vi "reset arm.vi"   [LabVIEW 2018]
uses:
  ARM angles.vi
types:
  T1 = enum16{"shoulder", "elbow", "wrist", "base", "gripper"}
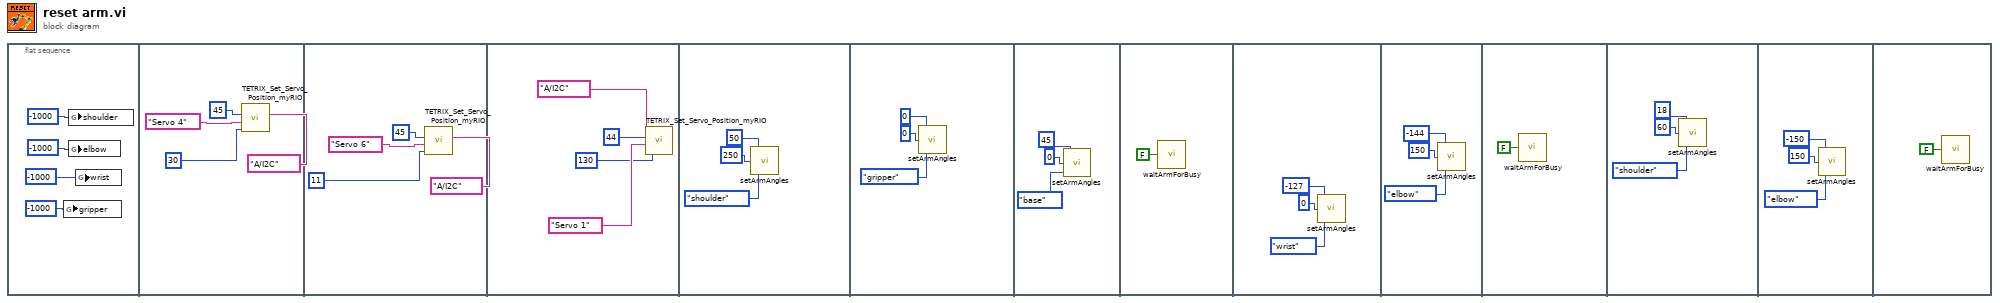
[diagram p0: block diagram]
diagram:
  n1 = flat-sequence {
    frame #0 {
      n2 = global write "ARM angles.vi" "gripper"(-1000 ("shoulder")) -> ()
      n3 = global write "ARM angles.vi" "shoulder"(-1000 ("shoulder")) -> ()
      n4 = global write "ARM angles.vi" "elbow"(-1000 ("shoulder")) -> ()
      n5 = global write "ARM angles.vi" "wrist"(-1000 ("shoulder")) -> ()
    }
    frame #1 {
      n6 = call <vilib>:"TETRIX_Set_Servo_Position_myRIO.vi"("myRIO MXP Port A/B"=tag "A/I2C", "Set Servo Position (0 - 180 degrees)"=u8 30, "Select Channel"="Servo 4", "Controller ID#  (I2C Address)"=u8 45) -> ()  [unwired: 3 in, 1 out]
    }
    frame #2 {
      n7 = call <vilib>:"TETRIX_Set_Servo_Position_myRIO.vi"("myRIO MXP Port A/B"=tag "A/I2C", "Set Servo Position (0 - 180 degrees)"=u8 11 ("Set Servo Position (0 - 180 degrees) 2"), "Select Channel"="Servo 6", "Controller ID#  (I2C Address)"=u8 45) -> ()  [unwired: 3 in, 1 out]
    }
    frame #3 {
      n8 = call <vilib>:"TETRIX_Set_Servo_Position_myRIO.vi"("myRIO MXP Port A/B"=tag "A/I2C", "Set Servo Position (0 - 180 degrees)"=u8 130, "Select Channel"="Servo 1", "Controller ID#  (I2C Address)"=u8 44) -> ()  [unwired: 3 in, 1 out]
    }
    frame #4 {
      n9 = call "setArmAngles.vi"("Enum"=T1."shoulder", "speed"=250, "angle"=50) -> ()  [unwired: 1 in]
    }
    frame #5 {
      n10 = call "setArmAngles.vi"("Enum"=T1."gripper", "speed"=0, "angle"=0) -> ()  [unwired: 1 in]
    }
    frame #6 {
      n11 = call "setArmAngles.vi"("Enum"=T1."base", "speed"=0, "angle"=45) -> ()  [unwired: 1 in]
    }
    frame #7 {
      n12 = call "waitArmForBusy.vi"("base"=FALSE) -> ()
    }
    frame #8 {
      n13 = call "setArmAngles.vi"("Enum"=T1."wrist", "speed"=0, "angle"=-127) -> ()  [unwired: 1 in]
    }
    frame #9 {
      n14 = call "setArmAngles.vi"("Enum"=T1."elbow", "speed"=150, "angle"=-144) -> ()  [unwired: 1 in]
    }
    frame #10 {
      n15 = call "waitArmForBusy.vi"("base"=FALSE) -> ()
    }
    frame #11 {
      n16 = call "setArmAngles.vi"("Enum"=T1."shoulder", "speed"=60, "angle"=18) -> ()  [unwired: 1 in]
    }
    frame #12 {
      n17 = call "setArmAngles.vi"("Enum"=T1."elbow", "speed"=150, "angle"=-150) -> ()  [unwired: 1 in]
    }
    frame #13 {
      n18 = call "waitArmForBusy.vi"("base"=FALSE) -> ()
    }
  }
